vi "Form Value-Connections Map.vi"(8 "error in (no error)":errorcluster, 11 "Channel States":T3) -> (0 "error out":errorcluster, 3 "Value-Connections Map":T1)   [LabVIEW 2017, in "Routing and Faulting System Explorer.lvlib"]
uses:
  Shared/Channel States.ctl
  Shared/Routing State.ctl
  Shared/Connection.ctl
  Shared/Value-Connections Map.ctl
  Routing and Faulting System Explorer.lvlib
  Shared/Routing and Faulting Shared.lvlib
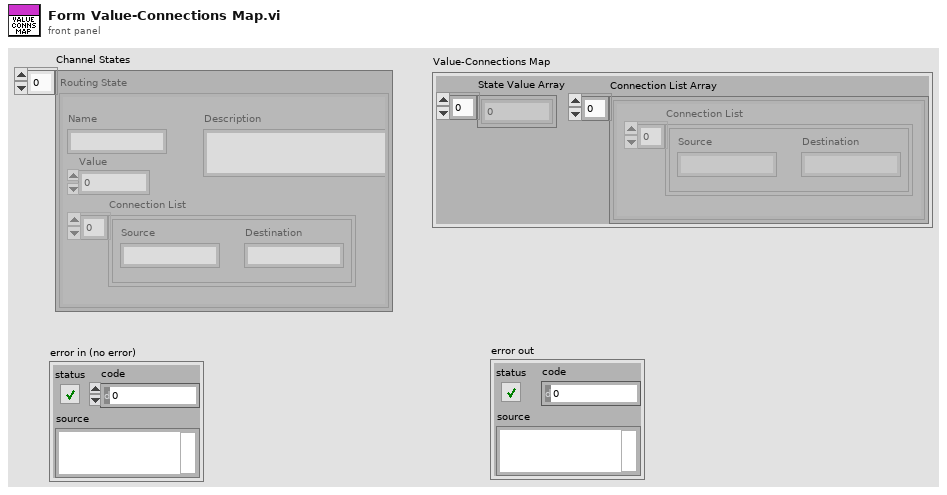
[diagram p1: front panel]
types:
  T1 = typedef "Routing and Faulting Shared.lvlib/Value-Connections Map.ctl" = cluster{"State Value Array":i32[], "Connection List Array":cluster{"Connection List":T2[]}[]}
  T2 = typedef "Routing and Faulting Shared.lvlib/Connection.ctl" = cluster{"Source":string, "Destination":string}
  T3 = typedef "Routing and Faulting Shared.lvlib/Channel States.ctl" = T4[]
  T4 = typedef "Routing and Faulting Shared.lvlib/Routing State.ctl" = cluster{"Name":string, "Description":string, "Value":i32, "Connection List":T2[]}
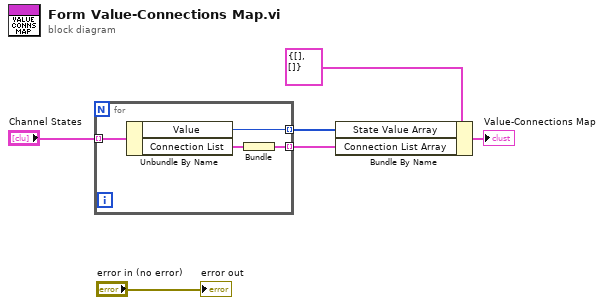
[diagram p0: block diagram]
diagram:
  n1 = for {
    tunnel: "Channel States" -> [w10] mode=indexing
    tunnel: [w9] -> w4 mode=indexing
    tunnel: [w7] -> w3 mode=indexing
    n2 = Unbundle By Name(w10) -> ("Value"=w9:i32, "Connection List"=w8:T2[])
    n3 = Bundle("Connection List"=w8) -> (w7:cluster{"Connection List":T2[]})  [unwired: 1 in]
  }
  n4 = Bundle By Name(cluster=T1 {"State Value Array"=[], "Connection List Array"=[]} ("Value-Connections Map"), "State Value Array"=w4, "Connection List Array"=w3) -> (→"Value-Connections Map":T1)
  "error out" <- "error in (no error)"
